vi "GetStringReference.vi"(8 "error in":errorcluster, 11 "String in":refnum<class "String.lvclass">) -> (0 "error out":errorcluster, 1 "String reference":refnum<vi>, 3 "String out":refnum<class "String.lvclass">)   [LabVIEW 2014, in "String.lvclass"]
uses:
  String.lvclass
  Generic/Generic.lvclass
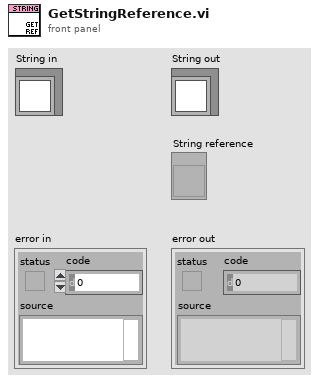
[diagram p1: front panel]
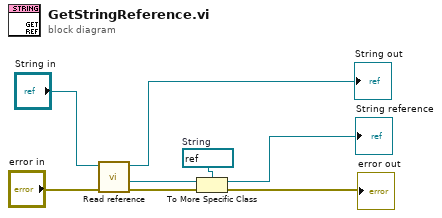
[diagram p0: block diagram]
diagram:
  w6 = refnum<vi> refnum  # String
  n1 = call "Read reference.vi"("error in"="error in", "GObject in"="String in") -> ("error out"=w7:errorcluster, "reference"=w8:refnum<vi>, "GObject out"=→"String out":refnum<class "String.lvclass">)  [unwired: 5 in]
  n2 = To More Specific Class(target class=w6, reference=w8, error in=w7) -> (specific class reference=→"String reference":refnum<vi>, error out=→"error out":errorcluster)
